vi "Dispense FN - ON - Mass Loss (SubVI).vi"(0 "Measured Mass (g)":dbl, 7 "State Change?":bool, 9 "Measure Dispense Delay (sec)":dbl, 11 "Settle Slope Sample Time (s)":dbl) -> (6 "Enable Dispense Measure":bool, 8 "Dispense Mass Loss":dbl, 10 "Dynamic SP Valid":bool)   [LabVIEW 2012]
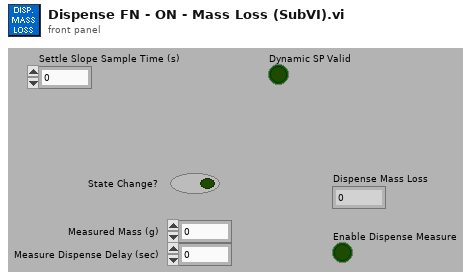
[diagram p1: front panel]
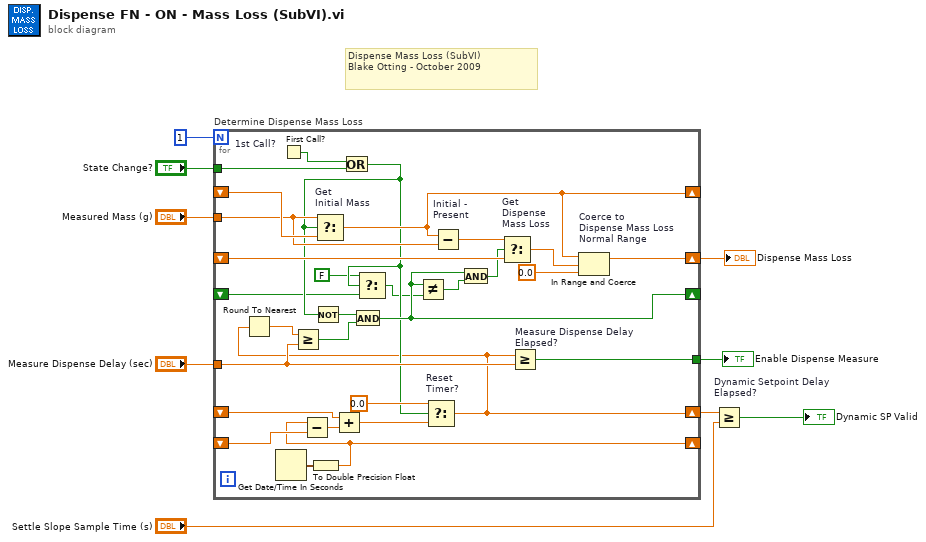
[diagram p0: block diagram]
diagram:
  # "Dispense Mass Loss (SubVI)\nBlake Otting - October 2009"
  n1 = for "Determine Dispense Mass Loss" {
    N: 1 -> [_]
    shift-right: [w11] -> w3
    shift-left: _ -> [w39]
    shift-right: [w30] -> _
    shift-left: _ -> [w38]
    tunnel: "Measured Mass (g)" -> [w26]
    shift-right: [w27] -> _
    shift-left: _ -> [w33]
    shift-right: [w25] -> w8
    shift-left: _ -> [w32]
    tunnel: [w21] -> w9
    tunnel: "State Change?" -> [w23]
    tunnel: "Measure Dispense Delay (sec)" -> [w19]
    shift-right: [w16] -> _
    shift-left: _ -> [w13]
    n2 = Get Date/Time In Seconds() -> (seconds since 1Jan1904=w37:timestamp)
    n3 = First Call? "1st Call?"() -> (First Call?: T/F=w10:bool)
    n4 = To Double Precision Float(number=w37) -> (double precision float=w30:dbl)
    n5 = Subtract(x=w30, y=w38) -> (x-y=w36:dbl)
    n6 = Add(x=w39, y=w36) -> (x+y=w35:dbl)
    n7 = Or(x=w10, y=w23) -> (x .or. y?=w15:bool)
    n8 = Not(x=w15) -> (.not. x?=w20:bool)
    n9 = Select "Get\nInitial Mass"(t=w26, s=w15, f=w33) -> (s? t:f=w27:dbl)
    n10 = Select(t=FALSE, s=w15, f=w13) -> (s? t:f=w12:bool)
    n11 = Select "Reset\nTimer?"(t=0.0, s=w15, f=w35) -> (s? t:f=w11:dbl)
    n12 = Round To Nearest(number=w11) -> (nearest integer value=w18:dbl)
    n13 = Greater Or Equal?(x=w18, y=w19) -> (x >= y?=w17:bool)
    n14 = And(x=w20, y=w17) -> (x .and. y?=w16:bool)
    n15 = Not Equal?(x=w16, y=w12) -> (x != y?=w24:bool)
    n16 = Subtract "Initial -\nPresent"(x=w27, y=w26) -> (x-y=w31:dbl)
    n17 = And(x=w16, y=w24) -> (x .and. y?=w22:bool)
    n18 = Select "Get\nDispense\nMass Loss"(t=w31, s=w22, f=w32) -> (s? t:f=w28:dbl)
    n19 = Greater Or Equal? "Measure Dispense Delay\nElapsed?"(x=w11, y=w19) -> (x >= y?=w21:bool)
    n20 = In Range and Coerce "Coerce to\nDispense Mass Loss \nNormal Range"(upper limit=w27, x=w28, lower limit=0.0) -> (coerced(x)=w25:dbl)  [unwired: 1 out]
  }
  "Dispense Mass Loss" <- w8
  "Enable Dispense Measure" <- w9
  n21 = Greater Or Equal? "Dynamic Setpoint Delay\nElapsed?"(x=w3, y="Settle Slope Sample Time (s)") -> (x >= y?=→"Dynamic SP Valid":bool)
